vi "ReadProperties.vi"(10 "Thing":string="Thing") -> (1 "Values":string[](array[string]), 2 "Names":string[](array[string]), 3 "All":string[][](array[string]))   [LabVIEW 2019]
panel:
  out "Type":string[](array[string])
  out "value":T1
  out "Comm":T2
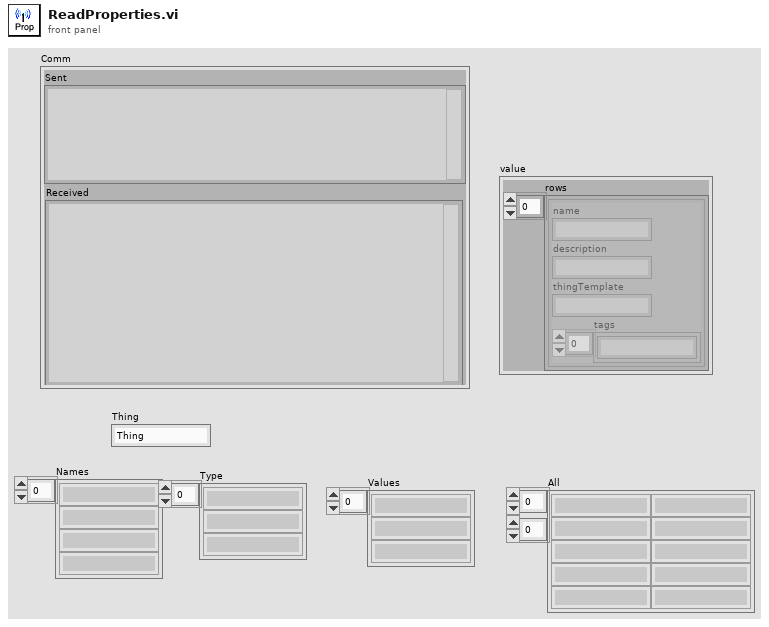
[diagram p1: front panel]
types:
  T1 = cluster{"rows":cluster{"name":string, "description":string, "thingTemplate":string, "tags":string[]}[]}
  T2 = cluster{"url":string, "sent headers":string, "sent body":string, "headers":string, "body":string, "Sent":string, "Received":string}
  T3 = cluster{"Name":string, "BaseURL":string, "AppKey":string, "Headers":string[], "Timeout":i32}
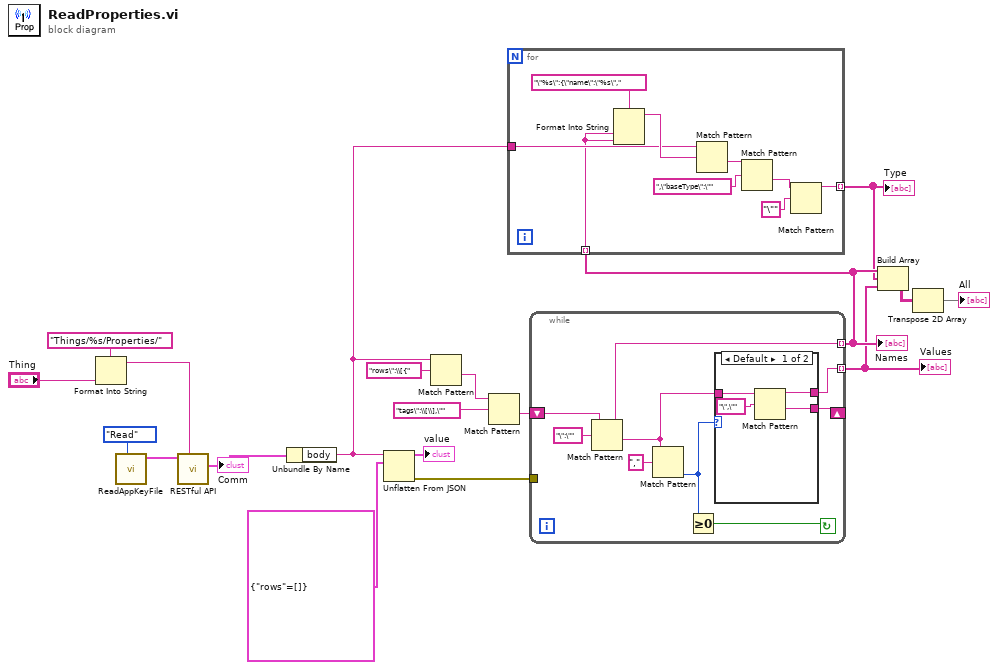
[diagram p0: block diagram]
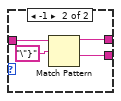
[diagram p2: hidden frame]
diagram:
  n1 = Format Into String(format string="Things/%s/Properties/" ("url"), "Thing") -> (resulting string=w8:string)  [unwired: 2 in, 1 out]
  n2 = call "ReadAppKeyFile.vi"("Task"=enum16{"Read", "Write"}."Read") -> ("Device Out"=w19:T3)  [unwired: 8 in, 2 out]
  n3 = call "RESTful API.vi"("url"=w8, "Device In"=w19) -> ("Comm"=w16:T2)  [unwired: 7 in, 2 out]
  "Comm" <- w16
  n4 = Unbundle By Name(w16) -> ("body"=w5:string)
  n5 = Unflatten From JSON(JSON string=w5, type and defaults=T1 {"rows"=[]} ("Cluster")) -> (value=→"value":T1, error out=w11:errorcluster)  [unwired: 5 in]
  n6 = Match Pattern(string=w5, regular expression="rows\":\\[{") -> (after substring=w13:string)  [unwired: 1 in, 3 out]
  n7 = Match Pattern(string=w13, regular expression="tags\":\\[\\],\"") -> (after substring=w12:string)  [unwired: 1 in, 3 out]
  n8 = while {
    shift-right: [w20] -> _
    shift-left: w12 -> [w27]
    tunnel: [w24] -> w4 mode=indexing
    tunnel: [w23] -> w2 mode=indexing
    tunnel: w11 -> [_]
    stop <- w25 continue-if-true
    n9 = Match Pattern(string=w27, regular expression="\":\"") -> (before substring=w24:string, after substring=w21:string)  [unwired: 1 in, 2 out]
    n10 = Match Pattern(string=w21, regular expression=",") -> (offset past match=w22:i32)  [unwired: 1 in, 3 out]
    n11 = Greater Or Equal To 0?(x=w22) -> (x >= 0?=w25:bool)
    n12 = case shown="Default" w22 {
      tunnel: w21 -> [w30 w35]
      tunnel: [w29 w34] -> w23
      tunnel: [w31 w33] -> w20
      frame Default {
        n13 = Match Pattern(string=w30, regular expression="\",\"") -> (before substring=w29:string, after substring=w31:string)  [unwired: 1 in, 2 out]
      }
      frame -1 {
        n14 = Match Pattern(string=w35, regular expression="\"}") -> (before substring=w34:string, after substring=w33:string)  [unwired: 1 in, 2 out]
      }
    }
  }
  "Names" <- w4
  "Values" <- w2
  n15 = for {
    tunnel: w5 -> [w43]
    tunnel: [w38] -> w3 mode=indexing
    tunnel: w4 -> [w37] mode=indexing
    n16 = Format Into String(format string="\"%s\":{\"name\":\"%s\"," ("regular expression"), w37, w37) -> (resulting string=w44:string)  [unwired: 2 in, 1 out]
    n17 = Match Pattern(string=w43, regular expression=w44) -> (after substring=w42:string)  [unwired: 1 in, 3 out]
    n18 = Match Pattern(string=w42, regular expression=",\"baseType\":\"") -> (after substring=w39:string)  [unwired: 1 in, 3 out]
    n19 = Match Pattern(string=w39, regular expression="\"") -> (before substring=w38:string)  [unwired: 1 in, 3 out]
  }
  "Type" <- w3
  n20 = Build Array(w4, w3, w2) -> (w7:string[][])
  n21 = Transpose 2D Array(2D array=w7) -> (transposed array=→"All":string[][])
